vi "ReadHBMFile.vi"(4 "error in (no error)":errorcluster, 6 "file path":path) -> (0 "error out":errorcluster, 2 "HBMWaveformsOut":waveform(dbl)[](graph))   [LabVIEW 2017]
panel:
  out "ChannelNames 2":string[](array[string])
  out "size(s) 3":i32
  out "WaveformComputational":waveform(dbl)[](graph)
  out "ChannelUnit 2":string[](array[string])
  out "size(s) 2":i32
  out "Unit":string
  out "Name":string
  out "ChannelUnit":string[](array[string])
  out "ChannelNames":string[](array[string])
  out "Waveform Graph 2":waveform(dbl)(graph)
  out "WaveformHardware":waveform(dbl)[](graph)
  out "size(s)":i32
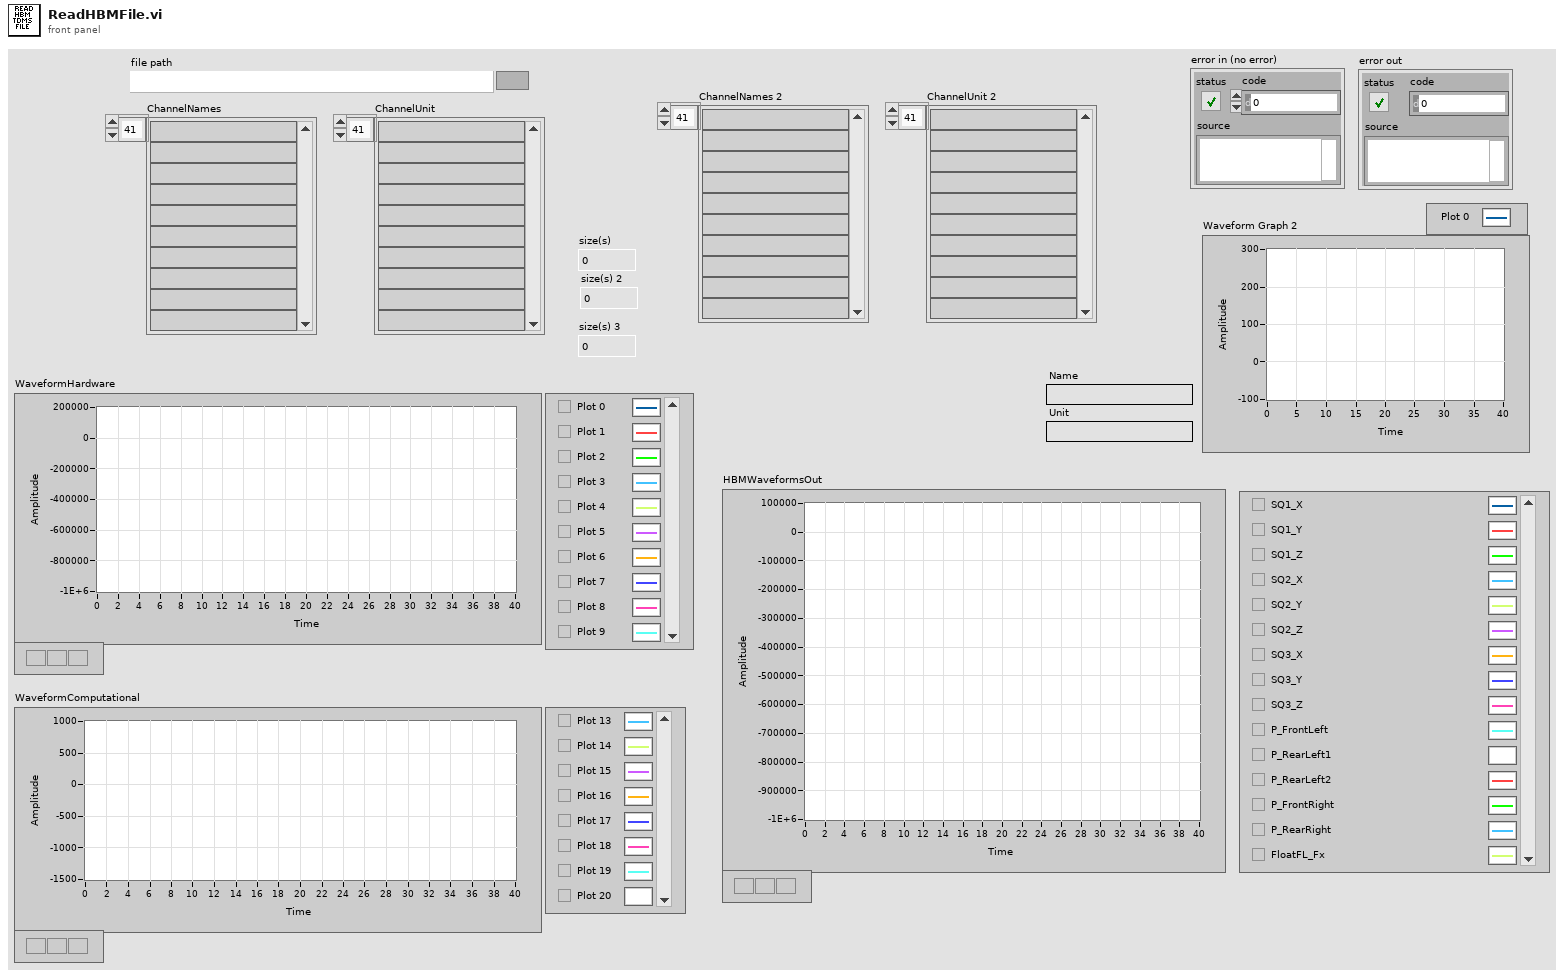
[diagram p1: front panel]
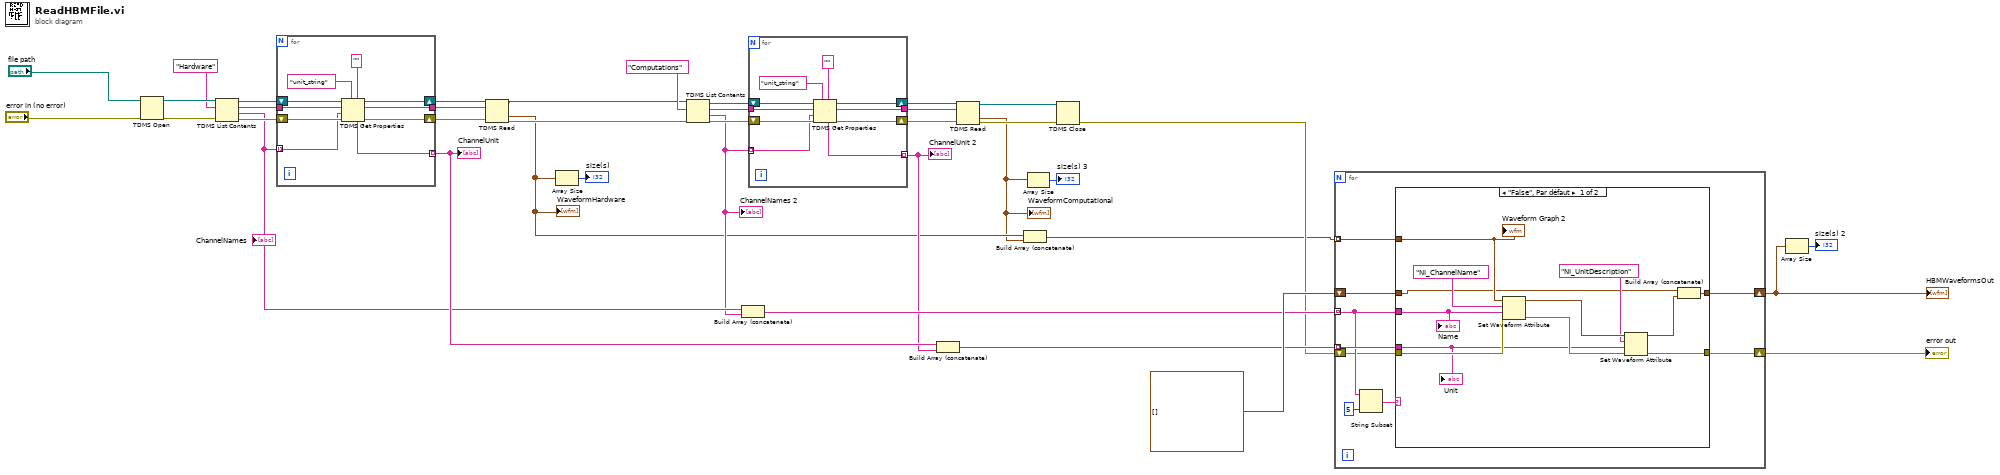
[diagram p0: block diagram]
diagram:
  n1 = TDMS Open(8:"error in (no error)", 11:"file path") -> (0:w35:errorcluster, 3:w34:refnum<k34>)  [unwired: 5 in]
  n2 = TDMS List Contents(4:w35, 6:"Hardware" ("group name"), 7:w34) -> (0:w32:errorcluster, 1:w5:string[], 2:w30:string, 3:w33:refnum<k34>)
  "ChannelNames" <- w5
  n3 = for {
    tunnel: w30 -> [w44]
    shift-right: [w46] -> w29
    shift-left: w33 -> [w48]
    shift-right: [w45] -> w28
    shift-left: w32 -> [w47]
    tunnel: w5 -> [w41] mode=indexing
    tunnel: [w40] -> w7 mode=indexing
    tunnel: [w39] -> w27
    n4 = TDMS Get Properties(5:"" ("property name"), 7:"unit_string" ("property name"), 8:w47, 9:w41, 10:w44, 11:w48) -> (0:w45:errorcluster, 2:w39:string, 3:w46:refnum<k34>, 4:w40:string)  [unwired: 2 out]
  }
  "ChannelUnit" <- w7
  n5 = TDMS Read(0:w29, 5:w27, 11:w28) -> (4:w11:refnum<k34>, 10:w3:waveform(dbl)[], 15:w12:errorcluster)  [unwired: 5 in, 3 out]
  "WaveformHardware" <- w3
  n6 = Array Size(array=w3) -> (size(s)=→"size(s)":i32)
  n7 = TDMS List Contents(4:w12, 6:"Computations" ("group name"), 7:w11) -> (0:w17:errorcluster, 1:w4:string[], 2:w19:string, 3:w16:refnum<k34>)
  "ChannelNames 2" <- w4
  n8 = Build Array (concatenate)(w5, w4) -> (w10:string[])
  n9 = for {
    tunnel: w19 -> [w54]
    shift-right: [w56] -> w20
    shift-left: w16 -> [w58]
    shift-right: [w55] -> w21
    shift-left: w17 -> [w57]
    tunnel: w4 -> [w51] mode=indexing
    tunnel: [w50] -> w6 mode=indexing
    tunnel: [w49] -> w22
    n10 = TDMS Get Properties(5:"" ("property name"), 7:"unit_string" ("property name"), 8:w57, 9:w51, 10:w54, 11:w58) -> (0:w55:errorcluster, 2:w49:string, 3:w56:refnum<k34>, 4:w50:string)  [unwired: 2 out]
  }
  "ChannelUnit 2" <- w6
  n11 = Build Array (concatenate)(w7, w6) -> (w9:string[])
  n12 = TDMS Read(0:w20, 5:w22, 11:w21) -> (4:w14:refnum<k34>, 10:w2:waveform(dbl)[], 15:w13:errorcluster)  [unwired: 5 in, 3 out]
  "WaveformComputational" <- w2
  n13 = Build Array (concatenate)(w3, w2) -> (w1:waveform(dbl)[])
  n14 = Array Size(array=w2) -> (size(s)=→"size(s) 3":i32)
  n15 = TDMS Close(8:w13, 11:w14) -> (0:w8:errorcluster)  [unwired: 1 out]
  n16 = for {
    tunnel: w1 -> [w67] mode=indexing
    tunnel: w10 -> [w64] mode=indexing
    tunnel: w9 -> [w66] mode=indexing
    shift-right: [w61] -> w23
    shift-left: waveform(dbl)[] [] -> [w60]
    shift-right: [w65] -> w26
    shift-left: w8 -> [w59]
    n17 = String Subset(string=w64, length (rest)=5 ("length (rest)")) -> (substring=w62:string)  [unwired: 1 in]
    n18 = case shown="\"False\", Par défaut" w62 {
      tunnel: w59 -> [w79 w80]
      tunnel: w67 -> [w78 _]
      tunnel: w66 -> [w73 _]
      tunnel: [w72 w80] -> w65
      tunnel: w64 -> [w71 _]
      tunnel: [w69 w81] -> w61
      tunnel: w60 -> [w68 w81]
      frame "False", Default {
        n19 = Set Waveform Attribute(4:w79, 5:w71, 6:"NI_ChannelName" ("name"), 7:w78) -> (0:w77:errorcluster, 3:w76:waveform(dbl))  [unwired: 1 out]
        n20 = Set Waveform Attribute(4:w77, 5:w73, 6:"NI_UnitDescription" ("name"), 7:w76) -> (0:w72:errorcluster, 3:w70:waveform(dbl))  [unwired: 1 out]
        n21 = Build Array (concatenate)(w68, w70) -> (w69:waveform(dbl)[])
        "Waveform Graph 2" <- w78
        "Name" <- w71
        "Unit" <- w73
      }
      frame "Temps" {
      }
    }
  }
  "HBMWaveformsOut" <- w23
  "error out" <- w26
  n22 = Array Size(array=w23) -> (size(s)=→"size(s) 2":i32)
